vi "2_AdvancedDemo_MHHisto.vi"() -> ()   [LabVIEW 2010]
uses:
  Types/MH_UIThread_Cmds.ctl
  _lib/PQ/MultiHarp/MH_InitInfo.ctl
  Types/MH_UIThread_Data.ctl
  Types/MH_InputChannel.ctl
  _lib/PQ/MultiHarp/MH_RefSource.ctl
  _lib/PQ/MultiHarp/mhlib_x86_x64_UIThread.llb/MH_DllPath_global.vi
  <vilib>/Utility/error.llb/DialogType.ctl
  _lib/PQ/MultiHarp/MH_LibVersion_global.vi
  _lib/PQ/MultiHarp/MH_MeasMode.ctl
panel:
  in  "Settings":bool=TRUE
  in  "Run continuously":bool=TRUE caption="Conti."
  in  "Start":bool
  in  "Scale":bool
  out "CountRates":i32[](graph)
  in  "HistoLength":i32(ring)=6 caption="Num Bins" items=["1024", "2048", "4096", "8192", "16384", "32768", "65536"]
  in  "OvlLevel":u32=100000 caption="Ovl.Level" min=1 step=1
  in  "StopOvl.":bool=TRUE
  in  "AcqTime":i32=1000 caption="Acqu.     ms" min=1 max=360000 step=1
  in  "Binning":i32(ring) caption="Resol.      ps" items=["80", "160", "320", "640", "1280", "2560", "5120", "10240", "20480", "40960", "81920", "163840", "327680", "655360", "1310720", "2621440", "5242880", "10485760", "20971520", "41943040", "83886080", "167772160", "335544320", "671088640", "1342177280", "2684354560"]
  in  "HistoOffset":i32 caption="Offset      ns" min=0 max=100000000 step=1
  out "HistoGraph":T1(graph)={0.0, "Resolution"=0.08, "Histogram"=[]}
  in  "SyncEdge":i32(ring) caption="Edge" items=["falling", "rising"]
  in  "SyncDivider":i32(ring)=3 caption="Divider" items=["1", "2", "4", "8", "16"]
  in  "SyncOffset":i32 caption="Offset      ps" min=-99999 max=99999 step=1
  in  "SyncLevel":i32=-50 caption="Level      mV" min=-1200 max=1200 step=1
  in  "Channels":T2[](array[typedef])=[{"Name"="Inp.Chan 1", "Enable"=TRUE, "Offset"=0, "Level"=-50, "Edge"=0}, {"Name"="Inp.Chan 2", "Enable"=TRUE, "Offset"=0, "Level"=-50, "Edge"=0}, {"Name"="Inp.Chan 3", "Enable"=TRUE, "Offset"=0, "Level"=-50, "Edge"=0}, {"Name"="Inp.Chan 4", "Enable"=TRUE, "Offset"=0, "Level"=-50, "Edge"=0}, {"Name"="Inp.Chan 5", "Enable"=TRUE, "Offset"=0, "Level"=-50, "Edge"=0}, {"Name"="Inp.Chan 6", "Enable"=TRUE, "Offset"=0, "Level"=-50, "Edge"=0}, {"Name"="Inp.Chan 7", "Enable"=TRUE, "Offset"=0, "Level"=-50, "Edge"=0}, {"Name"="Inp.Chan 8", "Enable"=TRUE, "Offset"=0, "Level"=-50, "Edge"=0}] {"Edge" items=["falling", "rising"]; "Offset" min=-99999 max=99999 step=80; "Level" min=-1200 max=1200 step=1}
  out "SyncRate":string="Sync Rate: 10000160 cps\n"
  out "OverFlow":bool caption="Overflow:"
  out "Status":string="Readout Rate: 7.4 Hz\t\tTotal Counts:\t\tCh. 1: 3766 cnts.\t\tCh. 2: 3766 cnts.\t\tCh. 3: 0 cnts.\t\tCh. 4: 0 cnts.\t\tCh. 5: 0 cnts.\t\tCh. 6: 0 cnts.\t\tCh. 7: 0 cnts.\t\tCh. 8: 0 cnts.\t\t"
  # "Histogram"
  # "Sync"
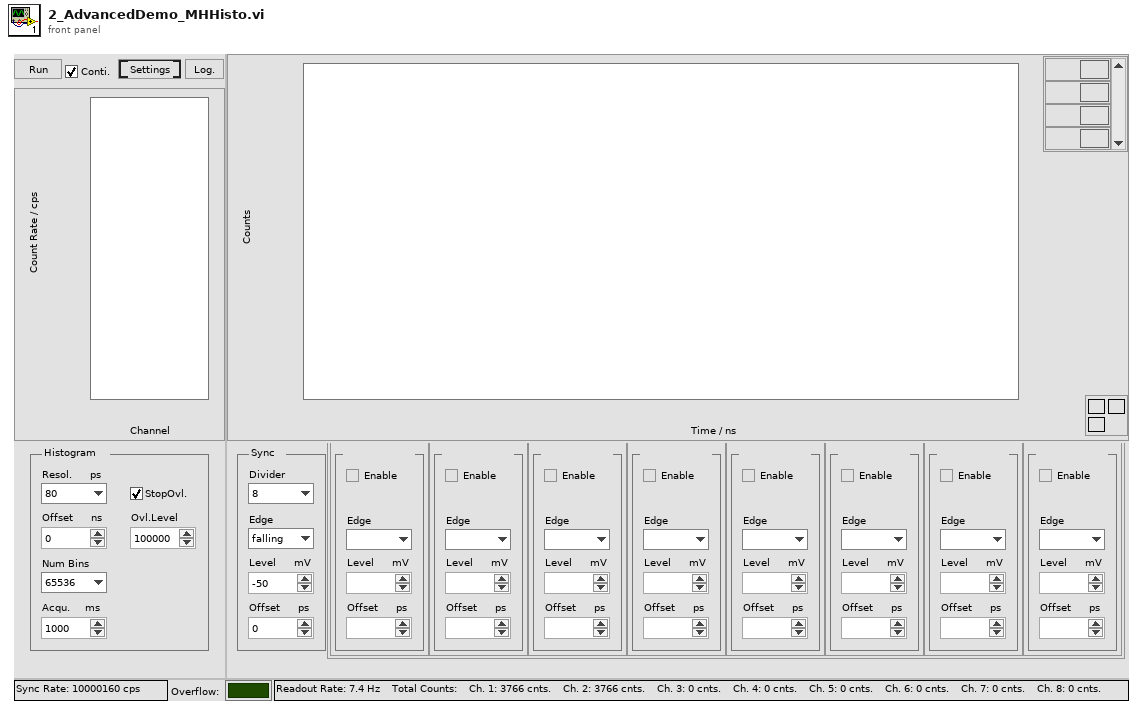
[diagram p1: front panel]
types:
  T1 = cluster{dbl, "Resolution":dbl, "Histogram":u32[][]}
  T2 = typedef "MH_InputChannel.ctl" = cluster{"Name":string, "Enable":bool, "Offset":i32, "Level":i32, "Edge":i32}
  T3 = typedef "MH_UIThread_Data.ctl" = cluster{"Init Info":T4, "DevIdx":i32, "SyncDivider":i32, "SyncOffset":i32, "SyncLevel":i32, "Channels":T2[], "CurrentChannels":i32[], "AcqTime":i32, "Binning":i32, "HistoOffset":i32, "HistoLen":i32, "StopOvl.":bool, "OvlLevel":u32, "SyncEdge":i32, "StartMeas":bool, "HistoLength":i32, "Resolution":dbl, "Run cont.":bool, "Status":string, "SyncRate":i32, "BitShift":i32, "HistoAcqTime":dbl}
  T4 = typedef "MH_InitInfo.ctl" = cluster{"Library Version":string, "Serial No.":string, "Model":string, "Partnum":string, "Version":string, "features":i32, "nchannels":i32, "Base Resolution":dbl, "Bin Steps":i32}
  T5 = typedef "MH_UIThread_Cmds.ctl" = enum16{"Idle", "Init", "SetInpChanEnable", "SetInpChanOffset", "SetInpChanTrg", "SetSyncDivider", "SetSyncTrg", "SetSyncOffset", "SetBinning", "SetHistoOffset", "SetHistoLen", "SetStopOvl", "SetBitShift", "SetHistoAcqTime", "GetRates", "GetAllRates", "StartMeas", "StopMeas", "AbortMeas", "GetResolution", "GetHistos", "GetAllHistos", "ReadFiFo", "WriteStatus", "Resize", "EnableControls", "DisableControls", "Error", "Exit"}
  T6 = enum8{"Enabled", "Disabled", "Disabled and Grayed Out"}
  T7 = typedef "MH_MeasMode.ctl" = i32
  T8 = typedef "MH_RefSource.ctl" = enum16{"INTERNAL", "EXTERNAL_10MHZ", "WR_MASTER_GENERIC", "WR_SLAVE_GENERIC", "WR_GRANDM_GENERIC", "EXTN_GPS_PPS", "EXTN_GPS_PPS_UART", "WR_MASTER_MHARP", "WR_SLAVE_MHARP", "WR_GRANDM_MHARP"}
  T9 = cluster{dbl, "Resolution":dbl, "Histograms":u32[][]}
  T10 = typedef "DialogType.ctl" = u16
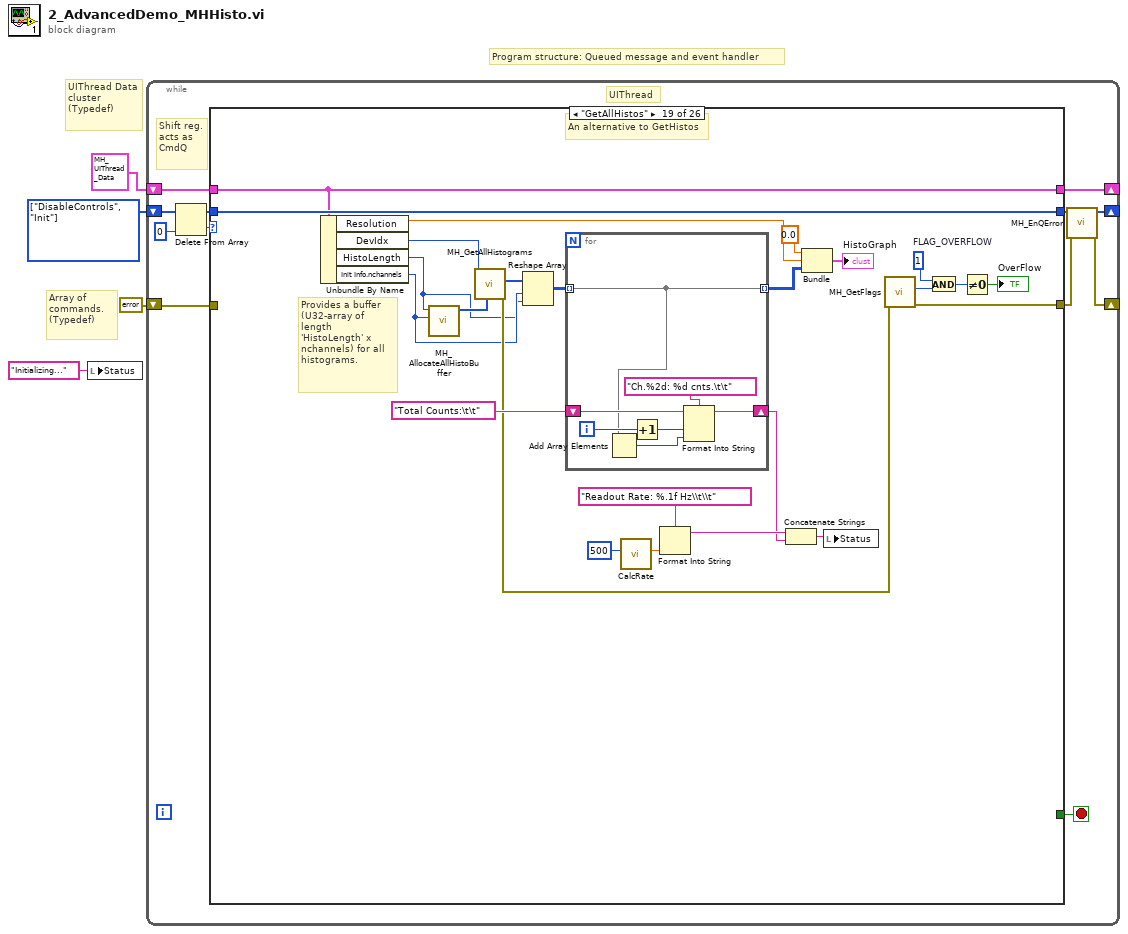
[diagram p0: block diagram]
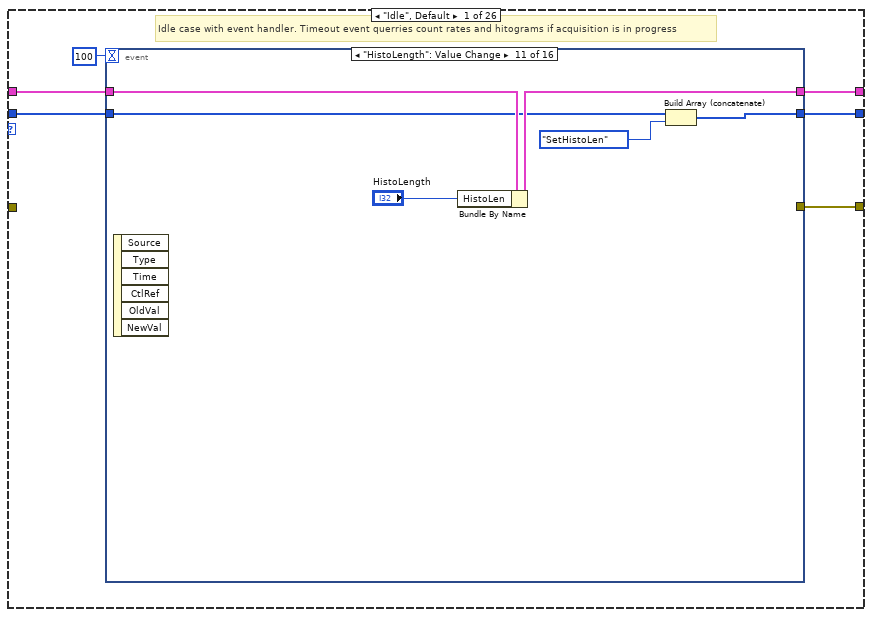
[diagram p2: hidden frame]
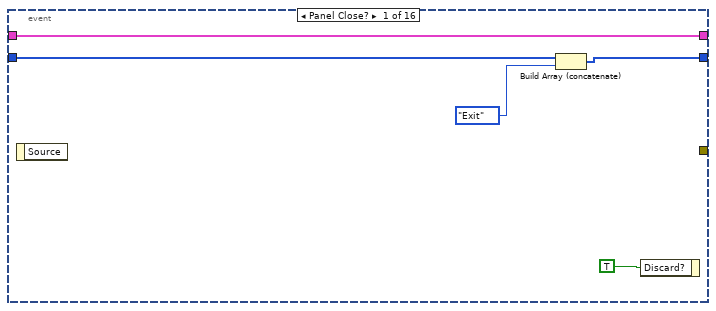
[diagram p3: hidden frame]
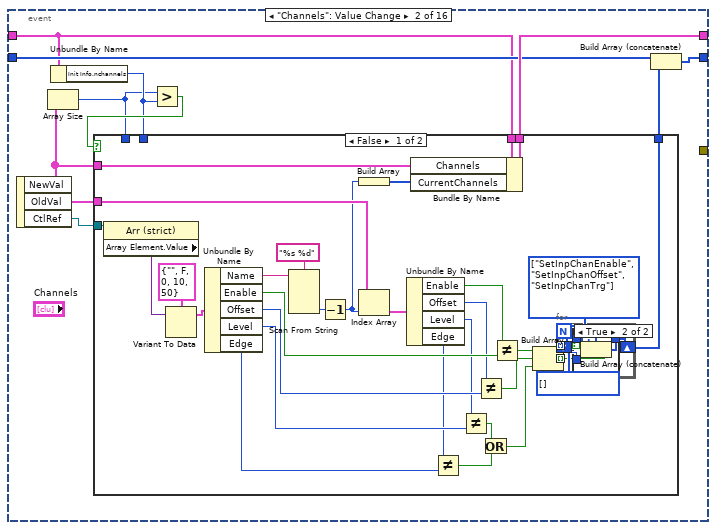
[diagram p4: hidden frame]
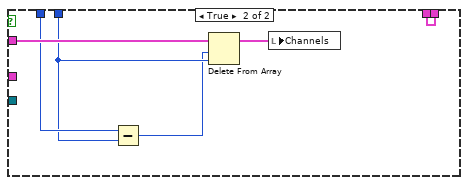
[diagram p6: hidden frame]
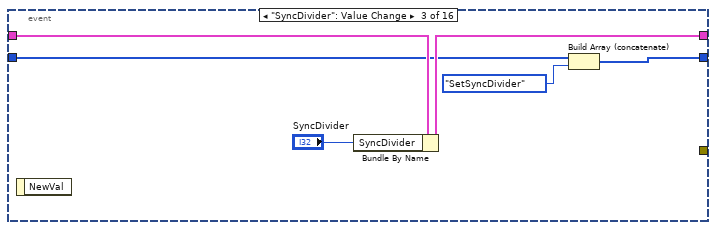
[diagram p7: hidden frame]
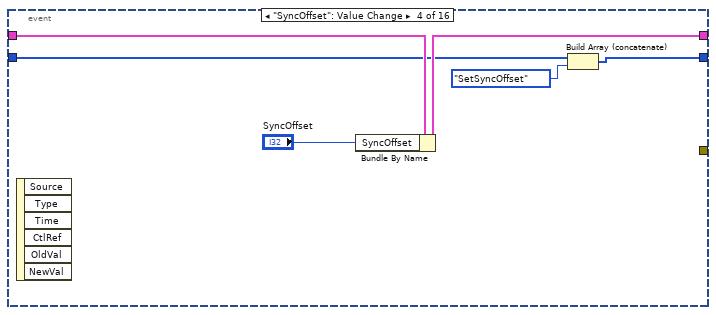
[diagram p8: hidden frame]
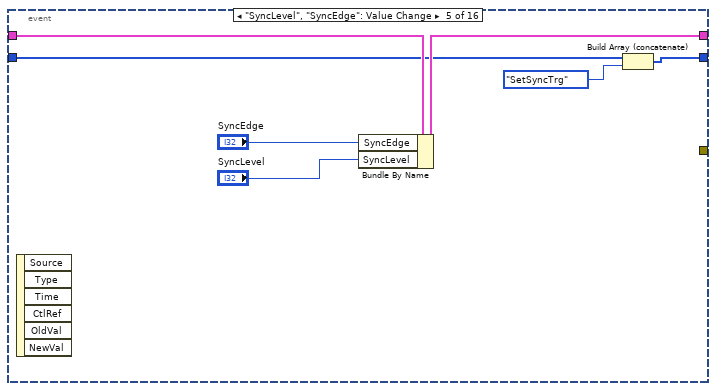
[diagram p9: hidden frame]
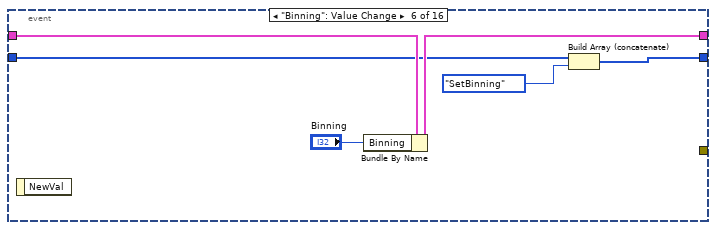
[diagram p10: hidden frame]
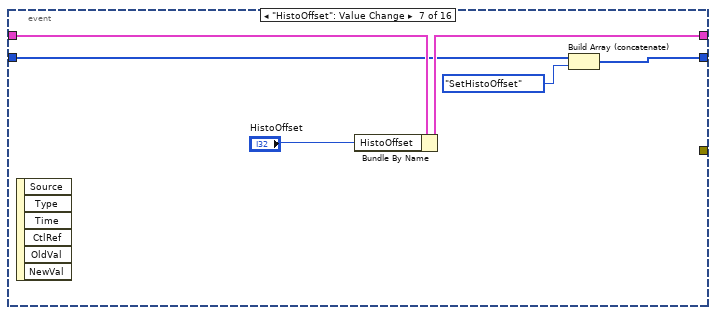
[diagram p11: hidden frame]
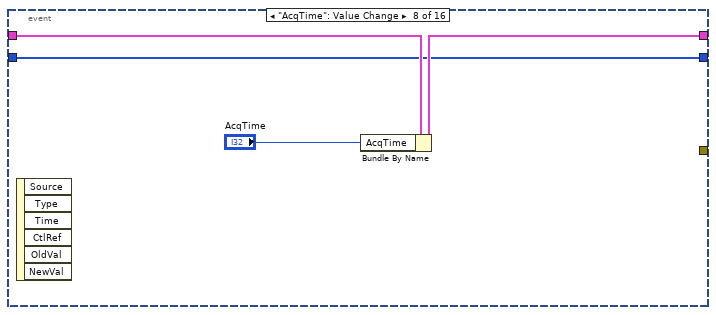
[diagram p12: hidden frame]
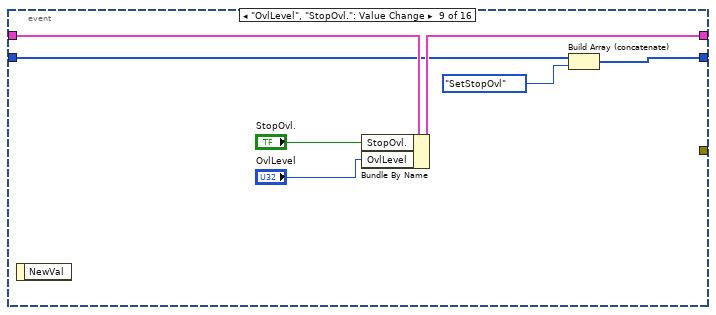
[diagram p13: hidden frame]
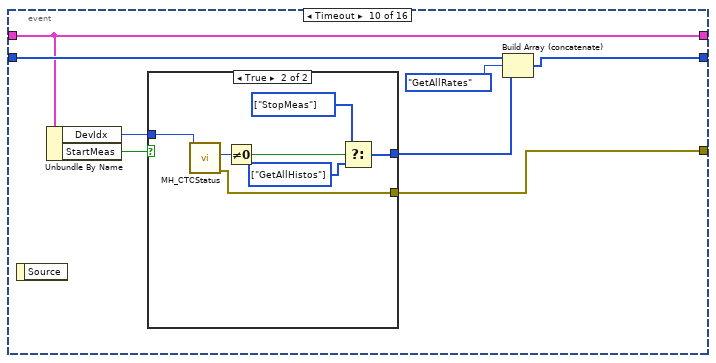
[diagram p14: hidden frame]
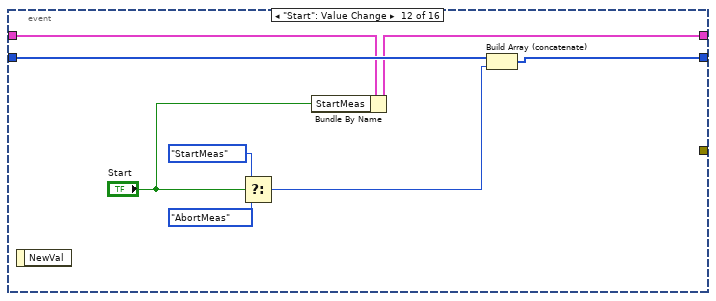
[diagram p16: hidden frame]
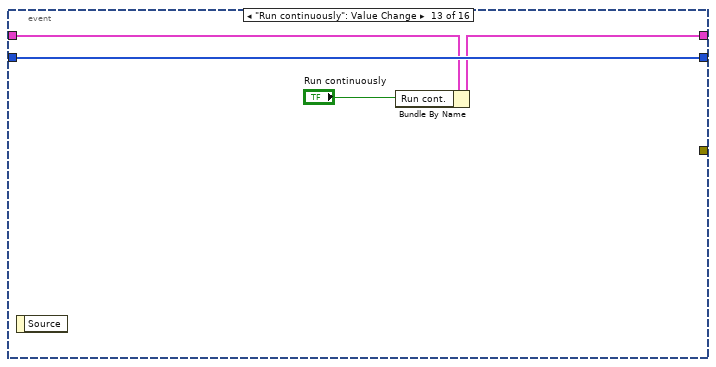
[diagram p17: hidden frame]
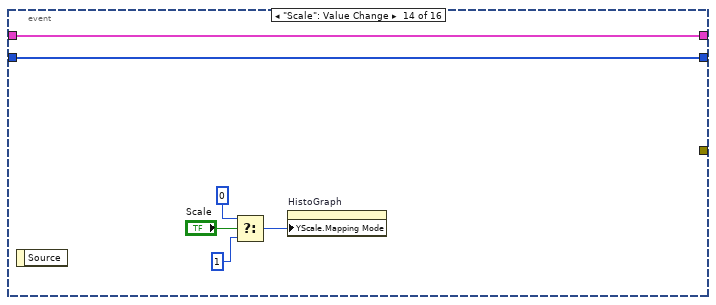
[diagram p18: hidden frame]
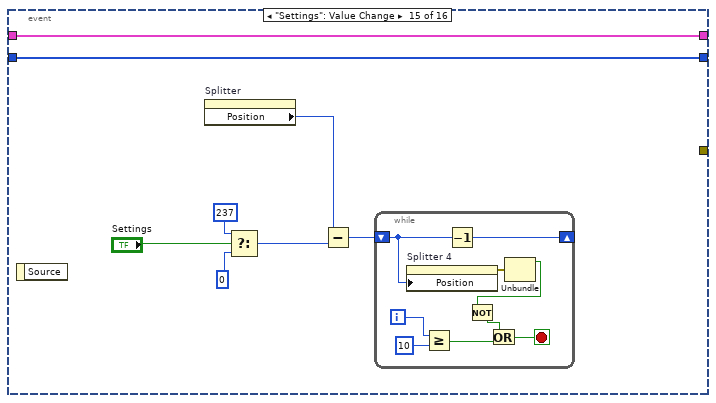
[diagram p19: hidden frame]
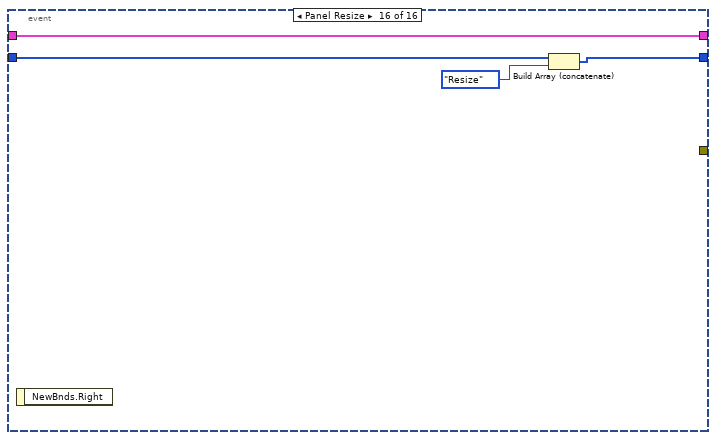
[diagram p20: hidden frame]
diagram:
  w3 = T5[] [enum."DisableControls", enum."Init"] items=["Idle", "Init", "SetInpChanEnable", "SetInpChanOffset", "SetInpChanTrg", "SetSyncDivider", "SetSyncTrg", "SetSyncOffset", "SetBinning", "SetHistoOffset", "SetHistoLen", "SetStopOvl", "SetBitShift", "SetHistoAcqTime", "GetRates", "GetAllRates", "StartMeas", "StopMeas", "AbortMeas", "GetResolution", "GetHistos", "GetAllHistos", "ReadFiFo", "WriteStatus", "Resize", "EnableControls", "DisableControls", "Error", "Exit"]
  # "Array of commands.\n(Typedef)"
  # "Program structure: Queued message and event handler"
  # "UIThread Data cluster\n(Typedef)"
  n1 = local write "Status"("Initializing..." ("Status")) -> ()
  n2 = while {
    shift-right: [w5] -> _
    shift-left: w3 -> [w12]
    shift-right: [w15] -> _
    shift-left: T3 {"Init Info"={"Library Version"="", "Serial No."="", "Model"="", "Partnum"="", "Version"="", "features"=0, "nchannels"=0, "Base Resolution"=0.0, "Bin Steps"=0}, "DevIdx"=0, "SyncDivider"=1, "SyncOffset"=0, "SyncLevel"=50, "Channels"=[], "CurrentChannels"=[], "AcqTime"=1, "Binning"=1, "HistoOffset"=1, "HistoLen"=1024, "StopOvl."=FALSE, "OvlLevel"=1024, "SyncEdge"=10, "StartMeas"=FALSE, "HistoLength"=0, "Resolution"=0.0, "Run cont."=FALSE, "Status"="", "SyncRate"=0, "BitShift"=0, "HistoAcqTime"=0.0} -> [w14]
    shift-right: [w7] -> _
    shift-left: errorcluster {"status"=FALSE, "code"=0, "source"=""} ("error IO") -> [w13]
    stop <- w16 stop-if-true
    # "Shift reg.\nacts as\nCmdQ"
    # "UIThread"
    n3 = Delete From Array(array=w12, index=0) -> (deleted portion=w10:T5, array with subset deleted=w9:T5[])  [unwired: 1 in]
    n4 = case shown="\"GetAllHistos\"" w10 {
      tunnel: [w22 w232 w255 w269 w283 w300 w309 w311 w318 w326 w334 w339 w350 w361 w376 w384 w398 w412 w437 w469 w493 w506 w513 w525 w531 w535] -> w6
      tunnel: [_ _ _ _ _ _ _ _ _ _ _ _ _ _ _ _ _ _ _ _ _ _ _ _ _ TRUE] -> w16
      tunnel: [w21 w212 w258 w272 w286 w302 w310 w315 w322 w327 w329 w340 w349 w360 w382 w387 w401 w408 w436 w468 w492 w494 w512 w524 w532 w538] -> w15
      tunnel: w14 -> [w20 w217 w258 w272 w286 w302 w310 w315 w322 w327 w330 w340 w349 w360 w382 w388 w402 w409 w436 w468 w492 w494 w512 w524 w532 w538]
      tunnel: [w17 w235 w256 w270 w284 w298 w308 w314 w321 w325 w333 w338 w343 w359 w381 w390 w404 w410 w434 w464 _ _ _ _ _ w536] -> w8
      tunnel: w13 -> [_ _ _ _ _ _ _ _ _ _ _ _ _ _ _ _ _ _ _ _ _ _ _ _ w533 _]
      tunnel: w9 -> [w19 w234 w255 w269 w283 w300 w309 w311 w317 w326 w334 w339 w350 w361 w377 w385 w399 w412 w437 w469 w493 w506 w513 w525 _ w535]
      frame "Idle", Default {
        # "Idle case with event handler. Timeout event querries count rates and hitograms if acquisition is in progress"
        n5 = event shown="[10] \"HistoLength\": Value Change" {
          selector: _ -> [_ _ _ _ _ _ _ _ _ _ _ _ _ _ _ _]
          dyn-events: _ -> [_ _ _ _ _ _ _ _ _ _ _ _ _ _ _ _]
          timeout: 100 -> [_ _ _ _ _ _ _ _ _ _ _ _ _ _ _ _]
          tunnel: [w23 w33 w84 w90 w97 w104 w110 w115 w121 w131 w142 w150 w158 w164 w172 w182] -> w22
          tunnel: [w26 w36 w88 w94 w101 w107 w113 w117 w124 w130 w145 w148 w156 w163 w171 w185] -> w21
          tunnel: w20 -> [w26 w32 w89 w95 w102 w108 w114 w118 w125 w130 w146 w149 w157 w163 w171 w185]
          tunnel: w19 -> [w25 w35 w86 w92 w99 w106 w112 w115 w123 w133 w144 w152 w158 w164 w172 w183]
          tunnel: [_ _ _ _ _ _ _ _ _ w126 _ _ _ _ _ _] -> w17
          event Panel Close? {
            n6 = event-data() -> ()  [unwired: 1 in, 1 out]
            n7 = Build Array (concatenate)(w25, MH_UIThread_Cmds."Exit") -> (w23:T5[])
            n8 = event-data("Discard?"=TRUE) -> ()  [unwired: 1 in, 1 out]
          }
          event "Channels": Value Change {
            n9 = event-data() -> ("NewVal"=w31:T2[], "OldVal"=w37:T2[], "CtlRef"=w38:refnum<vi>)  [unwired: 1 in]
            n10 = Array Size(array=w31) -> (size(s)=w28:i32)
            n11 = Unbundle By Name(w32) -> ("Init Info.nchannels"=w29:i32)
            n12 = Greater?(x=w28, y=w29) -> (0:w30:bool)
            n13 = case shown="False" w30 {
              tunnel: w38 -> [w69 _]
              tunnel: w37 -> [w63 _]
              tunnel: [w46 w83] -> w36
              tunnel: [w44 _] -> w34
              tunnel: w32 -> [w41 w83]
              tunnel: w31 -> [w40 w82]
              tunnel: w29 -> [_ w80]
              tunnel: w28 -> [_ w81]
              frame False {
                w39 = T5[] [] items=["Idle", "Init", "SetInpChanEnable", "SetInpChanOffset", "SetInpChanTrg", "SetSyncDivider", "SetSyncTrg", "SetSyncOffset", "SetBinning", "SetHistoOffset", "SetHistoLen", "SetStopOvl", "SetBitShift", "SetHistoAcqTime", "GetRates", "GetAllRates", "StartMeas", "StopMeas", "AbortMeas", "GetResolution", "GetHistos", "GetAllHistos", "ReadFiFo", "WriteStatus", "Resize", "EnableControls", "DisableControls", "Error", "Exit"] ("Array")
                w47 = T5[] [enum."SetInpChanEnable", enum."SetInpChanOffset", enum."SetInpChanTrg"] items=["Idle", "Init", "SetInpChanEnable", "SetInpChanOffset", "SetInpChanTrg", "SetSyncDivider", "SetSyncTrg", "SetSyncOffset", "SetBinning", "SetHistoOffset", "SetHistoLen", "SetStopOvl", "SetBitShift", "SetHistoAcqTime", "GetRates", "GetAllRates", "StartMeas", "StopMeas", "AbortMeas", "GetResolution", "GetHistos", "GetAllHistos", "ReadFiFo", "WriteStatus", "Resize", "EnableControls", "DisableControls", "Error", "Exit"]
                n14 = property class="Arr (strict)"(reference=w69) -> ("Array Element.Value"=w68:variant)  [unwired: 1 in, 2 out]
                n15 = Variant To Data(Variant=w68, type=T2 {"Name"="", "Enable"=FALSE, "Offset"=0, "Level"=10, "Edge"=50} ("Channel")) -> (data=w45:cluster{})  [unwired: 1 in, 1 out]
                n16 = Unbundle By Name(w45) -> ("Name"=w66:string, "Enable"=w60:bool, "Offset"=w58:i32, "Level"=w56:i32, "Edge"=w54:i32)
                n17 = Scan From String(format string="%s %d", input string=w66) -> (output 2=w64:i32)  [unwired: 5 in, 3 out]
                n18 = Decrement(x=w64) -> (x-1=w43:i32)
                n19 = Build Array(w43) -> (w42:i32[])
                n20 = Index Array(array=w63, index=w43) -> (element=w62:T2)
                n21 = Unbundle By Name(w62) -> ("Enable"=w61:bool, "Offset"=w59:i32, "Level"=w57:i32, "Edge"=w55:i32)
                n22 = Bundle By Name(cluster=w41, "Channels"=w40, "CurrentChannels"=w42) -> (w46:T3)
                n23 = Not Equal?(x=w55, y=w54) -> (x != y?=w49:bool)
                n24 = Not Equal?(x=w57, y=w56) -> (x != y?=w50:bool)
                n25 = Not Equal?(x=w59, y=w58) -> (x != y?=w52:bool)
                n26 = Or(x=w50, y=w49) -> (x .or. y?=w48:bool)
                n27 = Not Equal?(x=w61, y=w60) -> (x != y?=w53:bool)
                n28 = Build Array(w53, w52, w48) -> (w51:bool[])
                n29 = for {
                  tunnel: w51 -> [w72] mode=indexing
                  tunnel: w47 -> [w73] mode=indexing
                  shift-right: [w70] -> w44
                  shift-left: w39 -> [w71]
                  n30 = case shown="True" w72 {
                    tunnel: w71 -> [w74 w76]
                    tunnel: w73 -> [_ w75]
                    tunnel: [w74 w77] -> w70
                    frame False {
                    }
                    frame True {
                      n31 = Build Array (concatenate)(w76, w75) -> (w77:T5[])
                    }
                  }
                }
              }
              frame True {
                n32 = Subtract(x=w81, y=w80) -> (x-y=w79:i32)
                n33 = Delete From Array(array=w82, length=w79, index=w80) -> (array with subset deleted=w78:T2[])  [unwired: 1 out]
                n34 = local write "Channels"(w78) -> ()
              }
            }
            n35 = Build Array (concatenate)(w35, w34) -> (w33:T5[])
          }
          event "SyncDivider": Value Change {
            n36 = event-data() -> ()  [unwired: 1 in, 1 out]
            n37 = Bundle By Name(cluster=w89, "SyncDivider"="SyncDivider") -> (w88:T3)
            n38 = Build Array (concatenate)(w86, MH_UIThread_Cmds."SetSyncDivider") -> (w84:T5[])
          }
          event "SyncOffset": Value Change {
            n39 = event-data() -> ()  [unwired: 1 in, 6 out]
            n40 = Bundle By Name(cluster=w95, "SyncOffset"="SyncOffset") -> (w94:T3)
            n41 = Build Array (concatenate)(w92, MH_UIThread_Cmds."SetSyncOffset") -> (w90:T5[])
          }
          event "SyncLevel", "SyncEdge": Value Change {
            n42 = event-data() -> ()  [unwired: 1 in, 6 out]
            n43 = Bundle By Name(cluster=w102, "SyncEdge"="SyncEdge", "SyncLevel"="SyncLevel") -> (w101:T3)
            n44 = Build Array (concatenate)(w99, MH_UIThread_Cmds."SetSyncTrg") -> (w97:T5[])
          }
          event "Binning": Value Change {
            n45 = event-data() -> ()  [unwired: 1 in, 1 out]
            n46 = Bundle By Name(cluster=w108, "Binning"="Binning") -> (w107:T3)
            n47 = Build Array (concatenate)(w106, MH_UIThread_Cmds."SetBinning") -> (w104:T5[])
          }
          event "HistoOffset": Value Change {
            n48 = event-data() -> ()  [unwired: 1 in, 6 out]
            n49 = Bundle By Name(cluster=w114, "HistoOffset"="HistoOffset") -> (w113:T3)
            n50 = Build Array (concatenate)(w112, MH_UIThread_Cmds."SetHistoOffset") -> (w110:T5[])
          }
          event "AcqTime": Value Change {
            n51 = event-data() -> ()  [unwired: 1 in, 6 out]
            n52 = Bundle By Name(cluster=w118, "AcqTime"="AcqTime") -> (w117:T3)
          }
          event "OvlLevel", "StopOvl.": Value Change {
            n53 = event-data() -> ()  [unwired: 1 in, 1 out]
            n54 = Bundle By Name(cluster=w125, "StopOvl."="StopOvl.", "OvlLevel"="OvlLevel") -> (w124:T3)
            n55 = Build Array (concatenate)(w123, MH_UIThread_Cmds."SetStopOvl") -> (w121:T5[])
          }
          event Timeout {
            n56 = event-data() -> ()  [unwired: 1 in, 1 out]
            n57 = Unbundle By Name(w130) -> ("DevIdx"=w128:i32, "StartMeas"=w129:bool)
            n58 = case shown="True" w129 {
              tunnel: w128 -> [_ w140]
              tunnel: [_ w138] -> w127
              tunnel: [_ w135] -> w126
              frame False {
              }
              frame True {
                w136 = T5[] [enum."GetAllHistos"] items=["Idle", "Init", "SetInpChanEnable", "SetInpChanOffset", "SetInpChanTrg", "SetSyncDivider", "SetSyncTrg", "SetSyncOffset", "SetBinning", "SetHistoOffset", "SetHistoLen", "SetStopOvl", "SetBitShift", "SetHistoAcqTime", "GetRates", "GetAllRates", "StartMeas", "StopMeas", "AbortMeas", "GetResolution", "GetHistos", "GetAllHistos", "ReadFiFo", "WriteStatus", "Resize", "EnableControls", "DisableControls", "Error", "Exit"]
                w137 = T5[] [enum."StopMeas"] items=["Idle", "Init", "SetInpChanEnable", "SetInpChanOffset", "SetInpChanTrg", "SetSyncDivider", "SetSyncTrg", "SetSyncOffset", "SetBinning", "SetHistoOffset", "SetHistoLen", "SetStopOvl", "SetBitShift", "SetHistoAcqTime", "GetRates", "GetAllRates", "StartMeas", "StopMeas", "AbortMeas", "GetResolution", "GetHistos", "GetAllHistos", "ReadFiFo", "WriteStatus", "Resize", "EnableControls", "DisableControls", "Error", "Exit"]
                n59 = call "MH_CTCStatus.vi"("devidx"=w140) -> ("error out"=w135:errorcluster, "ctcstatus"=w139:i32)  [unwired: 8 in, 1 out]
                n60 = Not Equal To 0?(x=w139) -> (x != 0?=w134:bool)
                n61 = Select(t=w137, s=w134, f=w136) -> (s? t:f=w138:T5[])
              }
            }
            n62 = Build Array (concatenate)(w133, MH_UIThread_Cmds."GetAllRates", w127) -> (w131:T5[])
          }
          event "HistoLength": Value Change {
            n63 = event-data() -> ()  [unwired: 1 in, 6 out]
            n64 = Bundle By Name(cluster=w146, "HistoLen"="HistoLength") -> (w145:T3)
            n65 = Build Array (concatenate)(w144, MH_UIThread_Cmds."SetHistoLen") -> (w142:T5[])
          }
          event "Start": Value Change {
            n66 = event-data() -> ()  [unwired: 1 in, 1 out]
            n67 = Select(t=MH_UIThread_Cmds."StartMeas", s="Start", f=MH_UIThread_Cmds."AbortMeas") -> (s? t:f=w151:T5)
            n68 = Bundle By Name(cluster=w149, "StartMeas"="Start") -> (w148:T3)
            n69 = Build Array (concatenate)(w152, w151) -> (w150:T5[])
          }
          event "Run continuously": Value Change {
            n70 = event-data() -> ()  [unwired: 1 in, 1 out]
            n71 = Bundle By Name(cluster=w157, "Run cont."="Run continuously") -> (w156:T3)
          }
          event "Scale": Value Change {
            n72 = event-data() -> ()  [unwired: 1 in, 1 out]
            n73 = Select(t=u8 0 ("Y Scale.Mapping Mode"), s="Scale", f=u8 1 ("Y Scale.Mapping Mode")) -> (s? t:f=w159:u8)
            n74 = property on="HistoGraph" class="WFGraph (strict)"("YScale.Mapping Mode"=w159) -> ()  [unwired: 2 in, 2 out]
          }
          event "Settings": Value Change {
            n75 = event-data() -> ()  [unwired: 1 in, 1 out]
            n76 = property on="Splitter" class="Splitter"() -> ("Position"=w170:i32)  [unwired: 2 in, 2 out]
            n77 = Select(t=237 ("PosT"), s="Settings", f=0 ("PosF")) -> (s? t:f=w167:i32)
            n78 = Subtract(x=w170, y=w167) -> (x-y=w166:i32)
            n79 = while {
              shift-right: [w181] -> _
              shift-left: w166 -> [w174]
              i -> [w180]
              stop <- w177 stop-if-true
              n80 = property on="Splitter 4" class="Splitter"("Position"=w174) -> (error out=w173:errorcluster)  [unwired: 2 in, 1 out]
              n81 = Greater Or Equal?(x=w180, y=10) -> (x >= y?=w178:bool)
              n82 = Decrement(x=w174) -> (x-1=w181:i32)
              n83 = Unbundle(w173) -> ("status"=w176:bool)  [unwired: 2 out]
              n84 = Not(x=w176) -> (.not. x?=w175:bool)
              n85 = Or(x=w175, y=w178) -> (x .or. y?=w177:bool)
            }
          }
          event Panel Resize {
            n86 = event-data() -> ()  [unwired: 1 in, 1 out]
            n87 = Build Array (concatenate)(w183, MH_UIThread_Cmds."Resize") -> (w182:T5[])
          }
        }
      }
      frame "Init" {
        w190 = T7 0 items=["HIST"=0, "T2"=2, "T3"=3]  # Mode
        w204 = MH_RefSource."INTERNAL"  # refsource
        w219 = TRUE ("Run cont.")
        w221 = FALSE ("StartMeas")
        w222 = u32 100000 ("OvlLevel")
        w223 = TRUE ("StopOvl.")
        w224 = 6 ("HistoLen")
        w225 = 1000 ("AcqTime")
        w226 = 0 ("HistoOffset")
        w227 = 0 ("Binning")
        w228 = -50 ("SyncLevel")
        w229 = 0 ("SyncZeroX")
        w230 = 0 ("SyncOffset")
        w231 = 3 ("SyncDivider")
        w233 = T5[] [enum."SetSyncDivider", enum."SetSyncOffset", enum."SetSyncTrg", enum."SetInpChanEnable", enum."SetInpChanOffset", enum."SetInpChanTrg", enum."SetBinning", enum."SetHistoOffset", enum."SetHistoLen", enum."SetStopOvl", enum."Resize", enum."EnableControls", enum."WriteStatus"] items=["Idle", "Init", "SetInpChanEnable", "SetInpChanOffset", "SetInpChanTrg", "SetSyncDivider", "SetSyncTrg", "SetSyncOffset", "SetBinning", "SetHistoOffset", "SetHistoLen", "SetStopOvl", "SetBitShift", "SetHistoAcqTime", "GetRates", "GetAllRates", "StartMeas", "StopMeas", "AbortMeas", "GetResolution", "GetHistos", "GetAllHistos", "ReadFiFo", "WriteStatus", "Resize", "EnableControls", "DisableControls", "Error", "Exit"]
        # "Init HW"
        # "Set path to mhlib.dll"
        # "Init all FP controls and corresponding copy in UIThread Data cluster"
        # "EnQ list of commands"
        # "Array with Inp.Chan."
        # "Initialization: 1. Init HW -> get # of channels -> make array for Inp.Channels\n2. Init all FP controls and corresponding fields in UIThread Data cluster\n3. EnQ list of commands for further initialization"
        n88 = call <vilib>:"Error Cluster From Error Code.vi"("is warning? (False)"=FALSE, "show call chain? (False)"=TRUE, "error message (\"\")"="DLL not found!" ("error message (\"\")"), "error code (0)"=5000) -> ("error out"=w205:errorcluster)  [unwired: 5 in]
        n89 = call "GetDLLPath.vi"("DllName_32bit"="MHLib.dll" ("name or relative path"), "DllName_64bit"="MHLib64.dll" ("name or relative path")) -> ("file exists?"=w207:bool, "DLLPath"=w208:path)  [unwired: 8 in]
        n90 = global write "MH_DllPath_global.vi" "DllPath"(w208) -> ()
        n91 = Build Array (concatenate)(w234, w233) -> (w232:T5[])
        n92 = Select(t=errorcluster {"status"=FALSE, "code"=0, "source"=""} ("error IO"), s=w207, f=w205) -> (s? t:f=w213:errorcluster)
        n93 = global read "MH_LibVersion_global.vi" "Library Version"() -> (w203:string)
        n94 = call "InitMH_UIThread.vi"("error in (no error)"=w213, "Mode"=w190, "refsource"=w204, "Library Version"=w203) -> ("error out"=w235:errorcluster, "Init Info"=w238:T4, "DevIdx"=w237:i32)  [unwired: 5 in]
        n95 = local write "SyncDivider"(w231) -> ()
        n96 = local write "SyncOffset"(w230) -> ()
        n97 = local write "SyncEdge"(w229) -> ()
        n98 = local write "SyncLevel"(w228) -> ()
        n99 = local write "Binning"(w227) -> ()
        n100 = local write "HistoOffset"(w226) -> ()
        n101 = local write "AcqTime"(w225) -> ()
        n102 = local write "HistoLength"(w224) -> ()
        n103 = local write "StopOvl."(w223) -> ()
        n104 = local write "OvlLevel"(w222) -> ()
        n105 = local write "Start"(w221) -> ()
        n106 = local write "Run continuously"(w219) -> ()
        n107 = Bundle By Name(cluster=w217, "DevIdx"=w237, "Init Info"=w238, "Status"="Initialized!") -> (w216:T3)
        n108 = Unbundle By Name(w216) -> ("Init Info.Bin Steps"=w215:i32, "Init Info.nchannels"=w192:i32, "Init Info.Base Resolution"=w197:dbl)
        n109 = Initialize Array(u32 0, w192, 1024 ("dimension size")) -> (w196:u32[][])
        n110 = Divide(x=w197, y=1000.0) -> (x/y=w198:dbl)
        n111 = call "MH_CalcBinningValues.vi"("Bin Steps"=w215) -> ("BinningValues"=w220:cluster{"String":string, "Value":i32}[])  [unwired: 10 in]
        n112 = property on="Binning" class="Ring (strict)"("StringsAndValues[]"=w220) -> ()  [unwired: 2 in, 2 out]
        n113 = Bundle(0.0, w198, w196) -> (w195:cluster{dbl, dbl, u32[][]})  [unwired: 1 in]
        n114 = for {
          N: w192 -> [_]
          tunnel: T2 {"Name"="", "Enable"=FALSE, "Offset"=0, "Level"=10, "Edge"=50} ("Channel") -> [w251]
          tunnel: [w250] -> w191 mode=indexing
          tunnel: [w240] -> w193 mode=indexing
          tunnel: w195 -> [w241]
          i -> [w240]
          # "Init values for Inp. Channels"
          n115 = Increment(x=w240) -> (x+1=w239:i32)
          n116 = Format Into String(format string="Inp.Chan %d", w239) -> (resulting string=w248:string)  [unwired: 2 in, 1 out]
          n117 = Format Into String(format string="Ch.%d", w239) -> (resulting string=w242:string)  [unwired: 2 in, 1 out]
          n118 = property on="HistoGraph" class="WFGraph (strict)"("Value"=w241, "Active Plot"=w240, "Plot.Plot Name"=w242) -> ()  [unwired: 2 in, 2 out]
          n119 = Bundle By Name(cluster=w251, "Name"=w248, "Enable"=TRUE, "Offset"=0, "Level"=-50 ("CFDZeroX"), "Edge"=0 ("CFDLevel")) -> (w250:T2)
        }
        n120 = local write "Channels"(w191) -> ()
        n121 = Bundle By Name(cluster=w216, "Channels"=w191, "CurrentChannels"=w193, "SyncDivider"=w231, "SyncOffset"=w230, "SyncEdge"=w229, "SyncLevel"=w228, "Binning"=w227, "HistoOffset"=w226, "AcqTime"=w225, "HistoLen"=w224, "StopOvl."=w223, "OvlLevel"=w222, "StartMeas"=w221, "Run cont."=w219) -> (w212:T3)
        n122 = property on="HistoGraph" class="WFGraph (strict)"("LegPlotMin"=u32 4 ("Legend:Plot Minimum")) -> ()  [unwired: 2 in, 2 out]
        n123 = property on="Settings" class="Bool (strict)"("Val(Sgnl)"=TRUE ("Value (Signaling)")) -> ()  [unwired: 2 in, 2 out]
        n124 = property on="Scale" class="Bool (strict)"("Val(Sgnl)"=FALSE ("Value (Signaling)")) -> ()  [unwired: 2 in, 2 out]
      }
      frame "SetInpChanEnable" {
        n125 = Unbundle By Name(w258) -> ("DevIdx"=w257:i32, "Channels"=w252:T2[], "CurrentChannels"=w253:i32[])
        n126 = for {
          tunnel: w257 -> [w265]
          shift-right: [w264] -> w256
          shift-left: errorcluster {"status"=FALSE, "code"=0, "source"=""} ("error out") -> [w263]
          tunnel: w253 -> [w259] mode=indexing
          tunnel: w252 -> [w262]
          n127 = Index Array(array=w262, index=w259) -> (element=w261:T2)
          n128 = Unbundle By Name(w261) -> ("Enable"=w260:bool)
          n129 = call "MH_SetInputChannelEnable.vi"("error in (no error)"=w263, "enable"=w260, "channel"=w259, "devidx"=w265) -> ("error out"=w264:errorcluster)  [unwired: 6 in, 1 out]
        }
      }
      frame "SetInpChanOffset" {
        n130 = Unbundle By Name(w272) -> ("DevIdx"=w271:i32, "Channels"=w266:T2[], "CurrentChannels"=w267:i32[])
        n131 = for {
          tunnel: w271 -> [w277]
          shift-right: [w274] -> w270
          shift-left: errorcluster {"status"=FALSE, "code"=0, "source"=""} ("error out") -> [w275]
          tunnel: w267 -> [w276] mode=indexing
          tunnel: w266 -> [w279]
          n132 = Index Array(array=w279, index=w276) -> (element=w278:T2)
          n133 = Unbundle By Name(w278) -> ("Offset"=w273:i32)
          n134 = call "MH_SetInputChannelOffset.vi"("error in (no error)"=w275, "Offset"=w273, "channel"=w276, "devidx"=w277) -> ("error out"=w274:errorcluster)  [unwired: 6 in, 1 out]
        }
      }
      frame "SetInpChanTrg" {
        n135 = Unbundle By Name(w286) -> ("DevIdx"=w285:i32, "Channels"=w280:T2[], "CurrentChannels"=w281:i32[])
        n136 = for {
          tunnel: w285 -> [w289]
          shift-right: [w291] -> w284
          shift-left: errorcluster {"status"=FALSE, "code"=0, "source"=""} ("error out") -> [w292]
          tunnel: w281 -> [w290] mode=indexing
          tunnel: w280 -> [w294]
          n137 = Index Array(array=w294, index=w290) -> (element=w293:T2)
          n138 = Unbundle By Name(w293) -> ("Level"=w288:i32, "Edge"=w287:i32)
          n139 = call "MH_SetInputEdgeTrg.vi"("channel"=w290, "error in (no error)"=w292, "edge"=w287, "level"=w288, "devidx"=w289) -> ("error out"=w291:errorcluster)  [unwired: 5 in, 1 out]
        }
      }
      frame "SetSyncDivider" {
        n140 = Unbundle By Name(w302) -> ("DevIdx"=w301:i32, "SyncDivider"=w297:i32)
        n141 = Power Of 2(x=w297) -> (2^x=w296:dbl)
        n142 = To Long Integer(number=w296) -> (32bit integer=w295:i32)
        n143 = call "MH_SetSyncDiv.vi"("SyncDivider"=w295, "devidx"=w301) -> ("error out"=w299:errorcluster)  [unwired: 8 in, 1 out]
        n144 = flat-sequence {
          tunnel: w299 -> [w303]
          tunnel: [w303] -> w298
          frame #0 {
            n145 = Wait (ms)(milliseconds to wait=u32 100) -> ()  [unwired: 1 out]
          }
        }
      }
      frame "SetSyncTrg" {
        n146 = Unbundle By Name(w310) -> ("DevIdx"=w307:i32, "SyncLevel"=w305:i32, "SyncEdge"=w306:i32)
        n147 = call "MH_SetSyncEdgeTrg.vi"("edge"=w306, "level"=w305, "devidx"=w307) -> ("error out"=w308:errorcluster)  [unwired: 7 in, 1 out]
      }
      frame "SetSyncOffset" {
        n148 = Unbundle By Name(w315) -> ("DevIdx"=w313:i32, "SyncOffset"=w312:i32)
        n149 = call "MH_SetSyncChannelOffset.vi"("Offset"=w312, "devidx"=w313) -> ("error out"=w314:errorcluster)  [unwired: 8 in, 1 out]
      }
      frame "SetBinning" {
        # "When binning is changed the new resolution is querried"
        n150 = Unbundle By Name(w322) -> ("DevIdx"=w320:i32, "Binning"=w319:i32)
        n151 = call "MH_SetBinning.vi"("Binning"=w319, "devidx"=w320) -> ("error out"=w321:errorcluster)  [unwired: 8 in, 1 out]
        n152 = Build Array (concatenate)(MH_UIThread_Cmds."GetResolution", w317) -> (w318:T5[])
      }
      frame "SetHistoOffset" {
        n153 = Unbundle By Name(w327) -> ("DevIdx"=w324:i32, "HistoOffset"=w323:i32)
        n154 = call "MH_SetOffset.vi"("Offset"=w323, "devidx"=w324) -> ("error out"=w325:errorcluster)  [unwired: 8 in, 1 out]
      }
      frame "SetHistoLen" {
        n155 = Unbundle By Name(w330) -> ("DevIdx"=w332:i32, "HistoLen"=w331:i32)
        n156 = call "MH_SetHistoLen.vi"("lencode"=w331, "devidx"=w332) -> ("error out"=w333:errorcluster, "actuallen"=w328:i32)  [unwired: 7 in, 1 out]
        n157 = Bundle By Name(cluster=w330, "HistoLength"=w328) -> (w329:T3)
      }
      frame "SetStopOvl" {
        n158 = Unbundle By Name(w340) -> ("DevIdx"=w337:i32, "StopOvl."=w336:bool, "OvlLevel"=w335:u32)
        n159 = call "MH_SetStopOverflow.vi"("stopcount"=w335, "StopOnOverflow"=w336, "devidx"=w337) -> ("error out"=w338:errorcluster)  [unwired: 7 in, 1 out]
      }
      frame "GetAllRates" {
        # "An alternative to GetRates"
        n160 = Unbundle By Name(w349) -> ("DevIdx"=w346:i32, "Init Info.nchannels"=w341:i32)
        n161 = call "MH_AllocateCntRateBuffer.vi"("NumChan"=w341) -> ("Buffer"=w342:i32[])  [unwired: 10 in]
        n162 = call "MH_GetAllCountRates.vi"("cntrates_buf"=w342, "devidx"=w346) -> ("error out"=w343:errorcluster, "cntrates"=→"CountRates":i32[], "syncrate"=w345:i32)  [unwired: 6 in, 1 out]
        n163 = Format Into String(format string="Sync Rate: %d cps\n", w345) -> (resulting string=→"SyncRate":string)  [unwired: 2 in, 1 out]
      }
      frame "GetRates" {
        # "An alternative to GetAllRates"
        n164 = Unbundle By Name(w360) -> ("Init Info.nchannels"=w355:i32, "Channels"=w357:T2[], "DevIdx"=w356:i32)
        n165 = call "MH_GetSyncRate.vi"("devidx"=w356) -> ("error out"=w353:errorcluster, "syncrate"=w352:i32)  [unwired: 8 in, 1 out]
        n166 = Format Into String(format string="Sync Rate: %d cps\n", w352) -> (resulting string=w354:string)  [unwired: 2 in, 1 out]
        n167 = for {
          N: w355 -> [_]
          tunnel: w356 -> [w367]
          tunnel: [w364] -> w351 mode=indexing
          shift-right: [w366] -> w359
          shift-left: w353 -> [w368]
          tunnel: w357 -> [w363] mode=indexing
          i -> [w365]
          n168 = Unbundle By Name(w363) -> ("Enable"=w362:bool)
          n169 = case shown="True" w362 {
            tunnel: w368 -> [w369 w374]
            tunnel: w367 -> [_ w373]
            tunnel: [w369 w372] -> w366
            tunnel: w365 -> [_ w371]
            tunnel: [_ w370] -> w364
            frame False {
            }
            frame True {
              n170 = call "MH_GetCountRate.vi"("error in (no error)"=w374, "Channel"=w371, "devidx"=w373) -> ("error out"=w372:errorcluster, "rate"=w370:i32)  [unwired: 6 in, 1 out]
            }
          }
        }
        n171 = local write "SyncRate"(w354) -> ()
        n172 = local write "CountRates"(w351) -> ()
      }
      frame "StartMeas" {
        n173 = Unbundle By Name(w382) -> ("AcqTime"=w378:i32, "DevIdx"=w379:i32)
        n174 = call "MH_ClearHistMem.vi"("devidx"=w379) -> ("error out"=w380:errorcluster)  [unwired: 9 in, 1 out]
        n175 = call "MH_StartMeas.vi"("error in (no error)"=w380, "tacq"=w378, "devidx"=w379) -> ("error out"=w381:errorcluster)  [unwired: 7 in, 1 out]
        n176 = Build Array (concatenate)(w377, MH_UIThread_Cmds."GetAllHistos") -> (w376:T5[])
      }
      frame "StopMeas" {
        n177 = Unbundle By Name(w388) -> ("Run cont."=w383:bool, "DevIdx"=w389:i32)
        n178 = call "MH_StopMeas.vi"("devidx"=w389) -> ("error out"=w390:errorcluster)  [unwired: 9 in, 1 out]
        n179 = case shown="True" w383 {
          tunnel: w388 -> [w394 w396]
          tunnel: [w393 w396] -> w387
          tunnel: [w391 w395] -> w386
          frame False {
            w391 = T5[] [enum."GetAllHistos"] items=["Idle", "Init", "SetInpChanEnable", "SetInpChanOffset", "SetInpChanTrg", "SetSyncDivider", "SetSyncTrg", "SetSyncOffset", "SetBinning", "SetHistoOffset", "SetHistoLen", "SetStopOvl", "SetBitShift", "SetHistoAcqTime", "GetRates", "GetAllRates", "StartMeas", "StopMeas", "AbortMeas", "GetResolution", "GetHistos", "GetAllHistos", "ReadFiFo", "WriteStatus", "Resize", "EnableControls", "DisableControls", "Error", "Exit"]
            w392 = FALSE ("StartMeas")
            n180 = Bundle By Name(cluster=w394, "StartMeas"=w392) -> (w393:T3)
            n181 = local write "Start"(w392) -> ()
          }
          frame True {
            w395 = T5[] [enum."GetAllHistos", enum."StartMeas"] items=["Idle", "Init", "SetInpChanEnable", "SetInpChanOffset", "SetInpChanTrg", "SetSyncDivider", "SetSyncTrg", "SetSyncOffset", "SetBinning", "SetHistoOffset", "SetHistoLen", "SetStopOvl", "SetBitShift", "SetHistoAcqTime", "GetRates", "GetAllRates", "StartMeas", "StopMeas", "AbortMeas", "GetResolution", "GetHistos", "GetAllHistos", "ReadFiFo", "WriteStatus", "Resize", "EnableControls", "DisableControls", "Error", "Exit"]
          }
        }
        n182 = Build Array (concatenate)(w385, w386) -> (w384:T5[])
      }
      frame "AbortMeas" {
        w400 = T5[] [enum."GetAllHistos"] items=["Idle", "Init", "SetInpChanEnable", "SetInpChanOffset", "SetInpChanTrg", "SetSyncDivider", "SetSyncTrg", "SetSyncOffset", "SetBinning", "SetHistoOffset", "SetHistoLen", "SetStopOvl", "SetBitShift", "SetHistoAcqTime", "GetRates", "GetAllRates", "StartMeas", "StopMeas", "AbortMeas", "GetResolution", "GetHistos", "GetAllHistos", "ReadFiFo", "WriteStatus", "Resize", "EnableControls", "DisableControls", "Error", "Exit"]
        w397 = FALSE ("StartMeas")
        n183 = Unbundle By Name(w402) -> ("DevIdx"=w403:i32)
        n184 = call "MH_StopMeas.vi"("devidx"=w403) -> ("error out"=w404:errorcluster)  [unwired: 9 in, 1 out]
        n185 = Bundle By Name(cluster=w402, "StartMeas"=w397) -> (w401:T3)
        n186 = local write "Start"(w397) -> ()
        n187 = Build Array (concatenate)(w399, w400) -> (w398:T5[])
      }
      frame "GetResolution" {
        # "Resolution in ns"
        # "Gets resolution in ps"
        # "Resolution is saved in UIThread Data cluster in ns"
        n188 = Unbundle By Name(w409) -> ("DevIdx"=w411:i32)
        n189 = call "MH_GetResolution.vi"("devidx"=w411) -> ("error out"=w410:errorcluster, "resolution"=w407:dbl)  [unwired: 8 in, 1 out]
        n190 = Divide(x=w407, y=1000.0) -> (x/y=w405:dbl)
        n191 = Bundle By Name(cluster=w409, "Resolution"=w405) -> (w408:T3)
      }
      frame "GetAllHistos" {
        w425 = 1  # FLAG_OVERFLOW
        # "Provides a buffer (U32-array of length 'HistoLength' x nchannels) for all histograms."
        # "An alternative to GetHistos"
        n192 = Unbundle By Name(w436) -> ("Resolution"=w435:dbl, "DevIdx"=w417:i32, "HistoLength"=w413:i32, "Init Info.nchannels"=w414:i32)
        n193 = call "MH_AllocateAllHistoBuffer.vi"("NumChan"=w414, "HistoLength"=w413) -> ("Buffer"=w416:u32[])  [unwired: 9 in]
        n194 = call "MH_GetAllHistograms.vi"("Chcount"=w416, "devidx"=w417) -> ("error out"=w415:errorcluster, "Histograms"=w419:u32[])  [unwired: 7 in, 1 out]
        n195 = Reshape Array(w419, w414, w413) -> (w418:u32[][])
        n196 = for {
          tunnel: [w438] -> w427 mode=indexing
          shift-right: [w440] -> w421
          shift-left: "Total Counts:\t\t" -> [w439]
          tunnel: w418 -> [w438] mode=indexing
          i -> [w444]
          n197 = Add Array Elements(numeric array=w438) -> (sum=w441:u32)
          n198 = Increment(x=w444) -> (x+1=w442:i32)
          n199 = Format Into String(format string="Ch.%2d: %d cnts.\t\t", initial string=w439, w442, w441) -> (resulting string=w440:string)  [unwired: 1 in, 1 out]
        }
        n200 = call "CalcRate.vi"("Refresh(ms)"=u32 500) -> ("Rate / Hz"=w433:dbl)  [unwired: 8 in, 2 out]
        n201 = Format Into String(format string="Readout Rate: %.1f Hz\\t\\t", w433) -> (resulting string=w431:string)  [unwired: 2 in, 1 out]
        n202 = Concatenate Strings(w431, w421) -> (w430:string)
        n203 = Bundle(0.0, "Resolution"=w435, "Histograms"=w427) -> (→"HistoGraph":T9)  [unwired: 1 in]
        n204 = local write "Status"(w430) -> ()
        n205 = call "MH_GetFlags.vi"("error in (no error)"=w415) -> ("error out"=w434:errorcluster, "flags"=w424:i32)  [unwired: 8 in, 1 out]
        n206 = And(x=w425, y=w424) -> (x .and. y?=w426:i32)
        n207 = Not Equal To 0?(x=w426) -> (x != 0?=→"OverFlow":bool)
      }
      frame "GetHistos" {
        w454 = 1  # FLAG_OVERFLOW
        # "Provides a buffer (U32-array of length 'HistoLength') for histograms."
        # "An alternative to GetAllHistos"
        n208 = Unbundle By Name(w468) -> ("Resolution"=w465:dbl, "Init Info.nchannels"=w447:i32, "Channels"=w448:T2[], "DevIdx"=w467:i32, "HistoLength"=w466:i32)
        n209 = call "MH_AllocateHistoBuffer.vi"("HistoLength"=w466) -> ("Buffer"=w459:u32[])  [unwired: 10 in]
        n210 = for {
          N: w447 -> [_]
          tunnel: w467 -> [w482]
          tunnel: [w479] -> w457 mode=indexing
          tunnel: w459 -> [w480]
          shift-right: [w481] -> w456
          shift-left: errorcluster {"status"=FALSE, "code"=0, "source"=""} ("error IO") -> [w473]
          shift-right: [w474] -> w450
          shift-left: "Total Counts:\t\t" -> [w472]
          tunnel: w448 -> [w471] mode=indexing
          i -> [w478]
          n211 = Unbundle By Name(w471) -> ("Enable"=w470:bool)
          n212 = case shown="True" w470 {
            tunnel: w482 -> [_ w490]
            tunnel: [w483 w489] -> w481
            tunnel: w480 -> [w484 w488]
            tunnel: [w484 w487] -> w479
            tunnel: w478 -> [_ w486]
            tunnel: w473 -> [w483 w485]
            frame False {
            }
            frame True {
              n213 = call "MH_GetHistogram.vi"("Chcount"=w488, "error in (no error)"=w485, "channel"=w486, "devidx"=w490) -> ("error out"=w489:errorcluster, "Histogram"=w487:u32[])  [unwired: 5 in, 1 out]
            }
          }
          n214 = Add Array Elements(numeric array=w479) -> (sum=w475:u32)
          n215 = Increment(x=w478) -> (x+1=w476:i32)
          n216 = Format Into String(format string="Ch.%2d: %d cnts.\t\t", initial string=w472, w476, w475) -> (resulting string=w474:string)  [unwired: 1 in, 1 out]
        }
        n217 = call "CalcRate.vi"("Refresh(ms)"=u32 500) -> ("Rate / Hz"=w463:dbl)  [unwired: 8 in, 2 out]
        n218 = Format Into String(format string="Readout Rate: %.1f Hz\\t\\t", w463) -> (resulting string=w461:string)  [unwired: 2 in, 1 out]
        n219 = Concatenate Strings(w461, w450) -> (w460:string)
        n220 = Bundle(0.0, "Resolution"=w465, "Histogram"=w457) -> (w445:T1)  [unwired: 1 in]
        n221 = local write "HistoGraph"(w445) -> ()
        n222 = local write "Status"(w460) -> ()
        n223 = call "MH_GetFlags.vi"("error in (no error)"=w456) -> ("error out"=w464:errorcluster, "flags"=w453:i32)  [unwired: 8 in, 1 out]
        n224 = And(x=w454, y=w453) -> (x .and. y?=w455:i32)
        n225 = Not Equal To 0?(x=w455) -> (x != 0?=w446:bool)
        n226 = local write "OverFlow"(w446) -> ()
      }
      frame "WriteStatus" {
        n227 = Unbundle By Name(w492) -> ("Status"=→"Status":string)
      }
      frame "Resize" {
        n228 = property on="Pane 3" class="Pane"() -> ("Width"=w499:u32)  [unwired: 2 in, 2 out]
        n229 = Subtract(x=w499, y=i16 100 ("b")) -> (x-y=w505:u32)
        n230 = Unbundle By Name(w494) -> ("Init Info.nchannels"=w502:i32)
        n231 = Quotient & Remainder(x=w505, y=i16 99 ("m")) -> (floor(x/y)=w504:u32)  [unwired: 1 out]
        n232 = In Range and Coerce(upper limit=w502, x=w504, lower limit=4) -> (coerced(x)=w503:u32)  [unwired: 1 out]
        n233 = Equal?(x=w502, y=w503) -> (x = y?=w501:bool)
        n234 = Not(x=w501) -> (.not. x?=w500:bool)
        n235 = property on="Channels" class="Arr (strict)"("HorizScroll"=w500, "Number of Columns"=w503, "Index Values"=u32[] [0]) -> ()  [unwired: 2 in, 2 out]
      }
      frame "EnableControls" {
        n236 = property class="VI"() -> ("Panel"=w510:refnum<vi>)  [unwired: 2 in, 2 out]
        n237 = property class="Pnl"(reference=w510) -> ("Controls[]"=w509:refnum<vi>[])  [unwired: 1 in, 2 out]
        n238 = property class="Pnl"(reference=w510) -> ("Decos[]"=w511:refnum<vi>[])  [unwired: 1 in, 2 out]
        n239 = for {
          tunnel: w511 -> [w515] mode=indexing
          tunnel: TRUE -> [w514]
          n240 = property class="Decor"(reference=w515, "Visible"=w514) -> ()  [unwired: 1 in, 2 out]
        }
        n241 = for {
          tunnel: w509 -> [w518] mode=indexing
          tunnel: T6."Enabled" ("Disabled") -> [w517]
          tunnel: [w516] -> _
          n242 = property class="Ctl"(reference=w518, "DisabledEnum"=w517) -> (error out=w516:errorcluster)  [unwired: 1 in, 1 out]
        }
      }
      frame "DisableControls" {
        n243 = property class="VI"() -> ("Panel"=w522:refnum<vi>)  [unwired: 2 in, 2 out]
        n244 = property class="Pnl"(reference=w522) -> ("Controls[]"=w521:refnum<vi>[])  [unwired: 1 in, 2 out]
        n245 = property class="Pnl"(reference=w522) -> ("Decos[]"=w523:refnum<vi>[])  [unwired: 1 in, 2 out]
        n246 = for {
          tunnel: w523 -> [w527] mode=indexing
          tunnel: FALSE -> [w526]
          n247 = property class="Decor"(reference=w527, "Visible"=w526) -> ()  [unwired: 1 in, 2 out]
        }
        n248 = for {
          tunnel: w521 -> [w530] mode=indexing
          tunnel: T6."Disabled and Grayed Out" ("Disabled") -> [w529]
          tunnel: [w528] -> _
          n249 = property class="Ctl"(reference=w530, "DisabledEnum"=w529) -> (error out=w528:errorcluster)  [unwired: 1 in, 1 out]
        }
      }
      frame "Error" {
        w531 = T5[] [enum."Exit"] items=["Idle", "Init", "SetInpChanEnable", "SetInpChanOffset", "SetInpChanTrg", "SetSyncDivider", "SetSyncTrg", "SetSyncOffset", "SetBinning", "SetHistoOffset", "SetHistoLen", "SetStopOvl", "SetBitShift", "SetHistoAcqTime", "GetRates", "GetAllRates", "StartMeas", "StopMeas", "AbortMeas", "GetResolution", "GetHistos", "GetAllHistos", "ReadFiFo", "WriteStatus", "Resize", "EnableControls", "DisableControls", "Error", "Exit"]
        w534 = T10 1 items=["no dialog", "OK message", "continue or stop message", "OK message + warnings", "continue/stop + warnings"] ("type of dialog (OK msg:1)")
        # "Error case: If an error occures the user is informed and the programm terminates. Add your own code to handle error events (e.g. exception lists, etc.)"
        n250 = call <vilib>:"Simple Error Handler.vi"("type of dialog (OK msg:1)"=w534, "error in (no error)"=w533) -> ()  [unwired: 3 in, 5 out]
      }
      frame "Exit" {
        n251 = Unbundle By Name(w538) -> ("DevIdx"=w537:i32)
        n252 = call "MH_CloseDevice.vi"("devidx"=w537) -> ("error out"=w536:errorcluster)  [unwired: 9 in, 1 out]
      }
    }
    n253 = call "MH_EnQError.vi"("error in (no error)"=w8, "Cmds_in"=w6) -> ("error out"=w7:errorcluster, "Cmds_out"=w5:T5[])  [unwired: 8 in]
  }
